vi "helloworld.vi"() -> ()   [LabVIEW 2018]
panel:
  out "Numeric":dbl
  out "String 2":string="Hello world!"
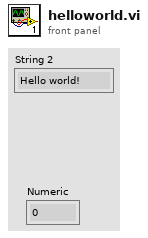
[diagram p1: front panel]
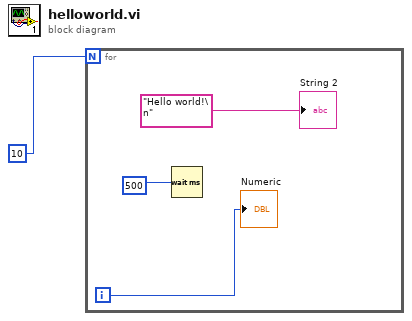
[diagram p0: block diagram]
diagram:
  n1 = for {
    N: 10 -> [_]
    i -> [w4]
    n2 = Wait (ms)(milliseconds to wait=500) -> ()  [unwired: 1 out]
    "Numeric" <- w4
    "String 2" <- "Hello world!\n" ("String")
  }
